vi "write keyword - integer.vi"(8 "error in (no error)":errorcluster, 9 "Value":i32, 10 "keyword":string, 11 "Simulated_Header in":refnum<class "Simulated_Header.lvclass">) -> (0 "error out":errorcluster, 3 "Simulated_Header out":refnum<class "Simulated_Header.lvclass">)   [LabVIEW 2018, in "Simulated_Header.lvclass"]
uses:
  Simulated_Header.lvclass
  Simulated_Header.lvclass/Simulated_Header.ctl
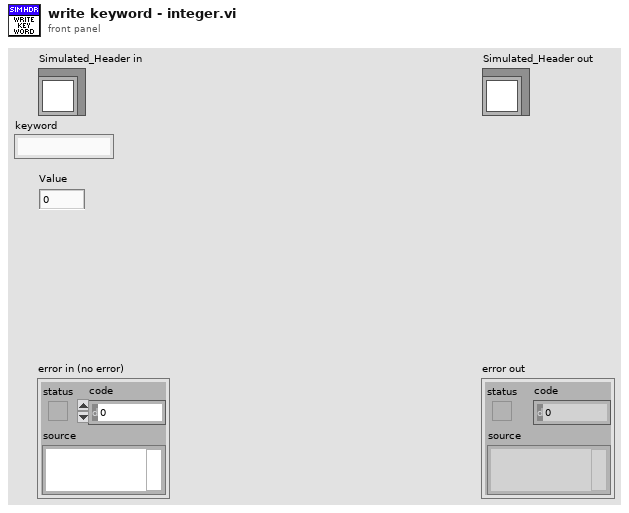
[diagram p1: front panel]
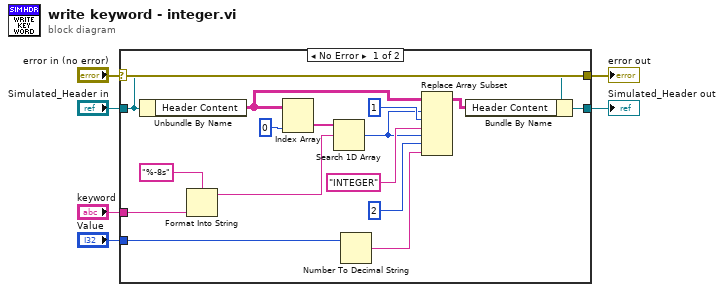
[diagram p0: block diagram]
diagram:
  n1 = case shown="No Error" "error in (no error)" {
    selector: "error in (no error)" -> [w22 w24]
    tunnel: [w22 w24] -> w5
    tunnel: [w16 w23] -> w3
    tunnel: "Simulated_Header in" -> [w17 w23]
    tunnel: "keyword" -> [w13 _]
    tunnel: "Value" -> [w8 _]
    frame No Error {
      n2 = Unbundle By Name(w17) -> ("Header Content"=w19:string[][])
      n3 = Format Into String(format string="%-8s", w13) -> (resulting string=w12:string)  [unwired: 2 in, 1 out]
      n4 = Index Array(array=w19, index (col)=0 ("disabled index (col)")) -> (element=w20:string[])  [unwired: 1 in]
      n5 = Search 1D Array(1D array=w20, element=w12) -> (index of element=w10:i32)  [unwired: 1 in]
      n6 = Number To Decimal String(number=w8) -> (decimal integer string=w7:string)  [unwired: 1 in]
      n7 = Replace Array Subset(array=w19, new element #1="INTEGER" ("new element/subarray"), index (row) #1=w10, index (col) #1=1 ("disabled index (col)"), new element #2=w7, index (row) #2=w10, index (col) #2=2 ("disabled index (col)")) -> (w15:string[][])
      n8 = Bundle By Name(cluster=w17, "Header Content"=w15) -> (w16:refnum<class "Simulated_Header.lvclass">)
    }
    frame Error {
    }
  }
  "error out" <- w5
  "Simulated_Header out" <- w3
